vi "Host Check File.vi"(6 "error":errorcluster, 8 "RT reference":refnum<vi>, 11 "File Path":path) -> (0 "File error":errorcluster, 3 "dup path":path, 4 "error out":errorcluster)   [LabVIEW 2023]
panel:
  in  "type specifier VI Refnum (for type only)":refnum<vi>
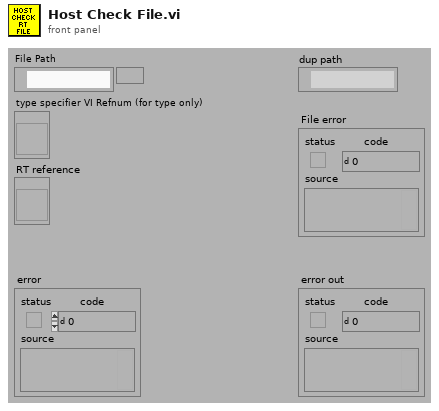
[diagram p1: front panel]
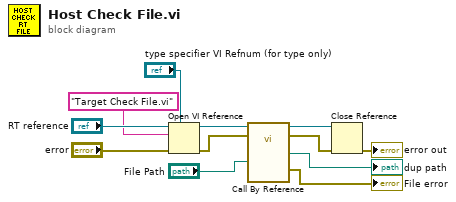
[diagram p0: block diagram]
diagram:
  n1 = Open VI Reference(type specifier VI Refnum (for type only)="type specifier VI Refnum (for type only)", application reference (local)="RT reference", vi path="Target Check File.vi", error in (no error)="error") -> (vi reference=w12:refnum<vi>, error out=w4:errorcluster)  [unwired: 2 in]
  n2 = call-by-ref "?"(reference=w12, error in=w4, "File Path"="File Path") -> (reference out=w3:refnum<vi>, error out=w2:errorcluster, "dup path"=→"dup path":path, 2:"error out"=→"File error":errorcluster)
  n3 = Close Reference(reference=w3, error in (no error)=w2) -> (error out=→"error out":errorcluster)
